vi "Read Report Folder.vi"(8 "error in (no error)":errorcluster, 11 "HtmlReportPlugin in":refnum<class "HtmlReportPlugin.lvclass">) -> (0 "error out":errorcluster, 2 "Report Folder":string, 3 "HtmlReportPlugin out":refnum<class "HtmlReportPlugin.lvclass">)   [LabVIEW 2015, in "HtmlReportPlugin.lvclass"]
uses:
  HtmlReportPlugin.lvclass
  HtmlReportPlugin.lvclass/HtmlReportPlugin.ctl
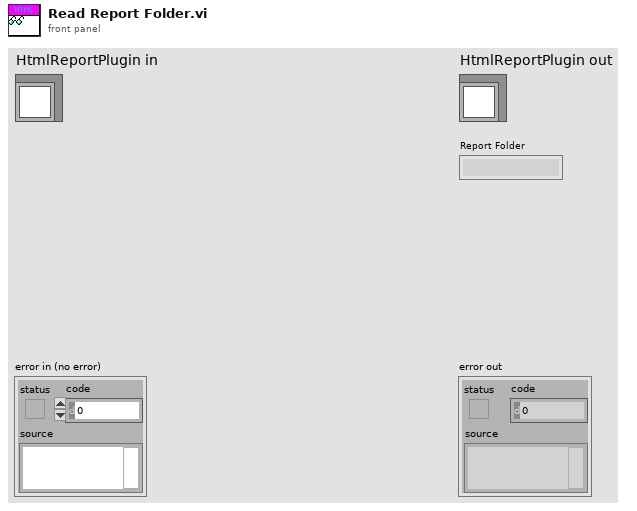
[diagram p1: front panel]
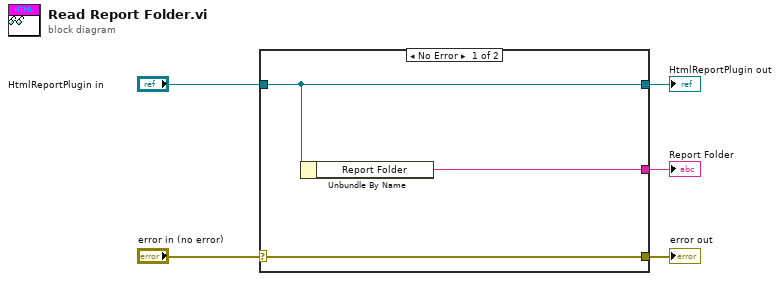
[diagram p0: block diagram]
diagram:
  n1 = case shown="No Error" "error in (no error)" {
    selector: "error in (no error)" -> [w8 w9]
    tunnel: [w8 w9] -> w4
    tunnel: [w7 w10] -> w2
    tunnel: "HtmlReportPlugin in" -> [w7 w10]
    tunnel: [w6 _] -> w1
    frame No Error {
      n2 = Unbundle By Name(w7) -> ("Report Folder"=w6:string)
    }
    frame Error {
    }
  }
  "error out" <- w4
  "HtmlReportPlugin out" <- w2
  "Report Folder" <- w1
